vi "Arms Controller.vi"(8 "error in":errorcluster) -> ()   [LabVIEW 2017]
doc: "This VI executes continuously carrying out the current operation and responding to updates or new operations. It will often contain the timing or control code that is difficult to place directly in TeleOp. This VI generally opens all sensors and motors and isolates the rest of the robot code from knowing how the operations are carried out."
uses:
  <vilib>/Rock Robotics/WPI/Framework/Completion Status.ctl
  Arms Setpoints.ctl
  Arms Operations.ctl
  <vilib>/Rock Robotics/SystemInterfaces/DIO/FPGA_DIOPWMChannel.ctl
  <vilib>/Rock Robotics/WPI/SafetyOutput/WPI_SafetyOutputConfigMenu.ctl
  <vilib>/Rock Robotics/SystemInterfaces/DIO/FPGA_DIOChannel.ctl
  <vilib>/Rock Robotics/WPI/MotorControl/WPI_MotorControlOpen VictorSP.vi
  <vilib>/Rock Robotics/WPI/Switch/WPI_SwitchOpenLimit.vi
  <vilib>/Rock Robotics/Network Tables/NT Write Boolean.vi
panel:
  in  "Interactive Values":T1
  out "Current\nCmd":string
  in  "Buttons":cluster{"Execute Cmd":bool, "Abort Cmd":bool}
  out "Command Timing":cluster{"Start Time (ms)":u32, "Iterations":i32}
  out "Status":T3
  # "Tip: It may be helpful to observe inputs and sensor values.\nYou may also want to display tuning or debugging controls."
  # "Interactive Command: You may fill in the settings for a command\nand schedule it with the Execute button. You can observe and abort\nany command while fine tuning the code for the controller."
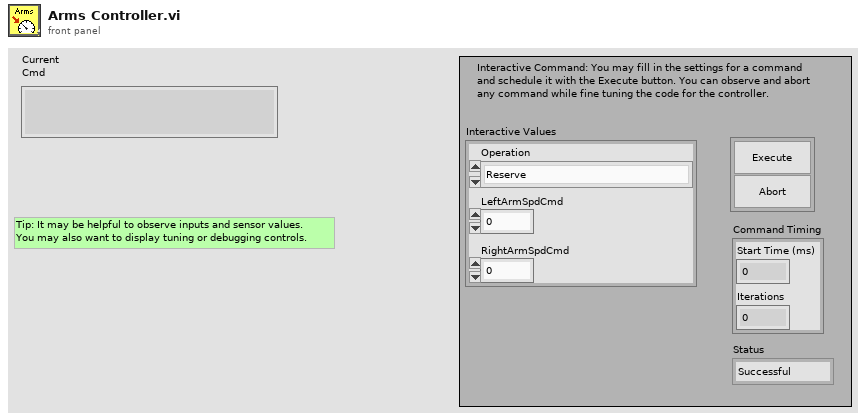
[diagram p1: front panel]
types:
  T1 = typedef "Arms Setpoints.ctl" = cluster{"Operation":T2, "LeftArmSpdCmd":dbl, "RightArmSpdCmd":dbl}
  T2 = typedef "Arms Operations.ctl" = enum16{"Reserve", "Read Current", "Immediate"}
  T3 = typedef "Completion Status.ctl" = enum16{"Successful", "Aborted", "Incomplete"}
  T4 = typedef "FPGA_DIOChannel.ctl" = enum8{"DIO 0", "DIO 1", "DIO 2", "DIO 3", "DIO 4", "DIO 5", "DIO 6", "DIO 7", "DIO 8", "DIO 9", "DIO MXP 0", "DIO MXP 1", "DIO MXP 2", "DIO MXP 3", "DIO MXP 4", "DIO MXP 5", "DIO MXP 6", "DIO MXP 7", "DIO MXP 8", "DIO MXP 9", "DIO MXP 10", "DIO MXP 11", "DIO MXP 12", "DIO MXP 13", "DIO MXP 14", "DIO MXP 15", "SPI Port CS1", "SPI Port CS2", "SPI Port CS3", "SPI Port MISO", "SPI Port MOSI", "Invalid"}
  T5 = typedef "FPGA_DIOPWMChannel.ctl" = enum8{"PWM 0", "PWM 1", "PWM 2", "PWM 3", "PWM 4", "PWM 5", "PWM 6", "PWM 7", "PWM 8", "PWM 9", "PWM MXP 0", "PWM MXP 1", "PWM MXP 2", "PWM MXP 3", "PWM MXP 4", "PWM MXP 5", "PWM MXP 6", "PWM MXP 7", "PWM MXP 8", "PWM MXP 9", "Invalid"}
  T6 = typedef "WPI_SafetyOutputConfigMenu.ctl" = enum16{"Enable", "Disable"}
  T7 = typedef "WPI_MotorControlDeviceRef.ctl" = cluster{"DeviceStatus":errorcluster, "Type":T8, "PWM":cluster{"PWM Channel":T5, "DeadBand":T9}, "CAN":cluster{"Device Number":u8, "SetOutput VI Ref":variant, "GetOutput VI Ref":variant, "Enable VI Ref":variant, "Disable VI Ref":variant, "Data":variant}, "Invert":bool, "DIO PWM":cluster{"PWM \"Enable\" Channel":T5, "DIOChannel":T4, "PWM Rate":dbl}}
  T8 = typedef "WPI_MotorControlType.ctl" = enum16{"PWM", "CAN", "DIO PWM"}
  T9 = typedef "WPI_PWMDeadband.ctl" = cluster{"Name":string, "maxPositivePwm":i32, "minPositivePwm":i32, "centerPwm":i32, "maxNegativePwm":i32, "minNegativePwm":i32, "angularRange":u16}
  T10 = typedef "WPI_SwitchDevRef.ctl" = cluster{"DevStatus":errorcluster, "DIO Channel":T4, "CntIndex":T11, "Normally Closed":bool}
  T11 = typedef "FPGA_CounterCtrSystemIndex.ctl" = enum8{"Ctr 0", "Ctr 1", "Ctr 2", "Ctr 3", "Ctr 4", "Ctr 5", "Ctr 6", "Ctr 7", "Invalid"}
  T12 = typedef "Command Status Info.ctl" = cluster{"Name":string, "Status":T3, "notifier out":T13}
  T13 = typedef "Completion Notifier.ctl" = refnum<notifier>
  T14 = cluster{"Current Command":T1, "Command Timing":cluster{"Start Time (ms)":u32, "Iterations":i32}, "Command Arguments":cluster{"Command Info":T12, "Description":string, "Default Command":T1, "queue out":refnum<queue>, "Subsystem Name":string}}
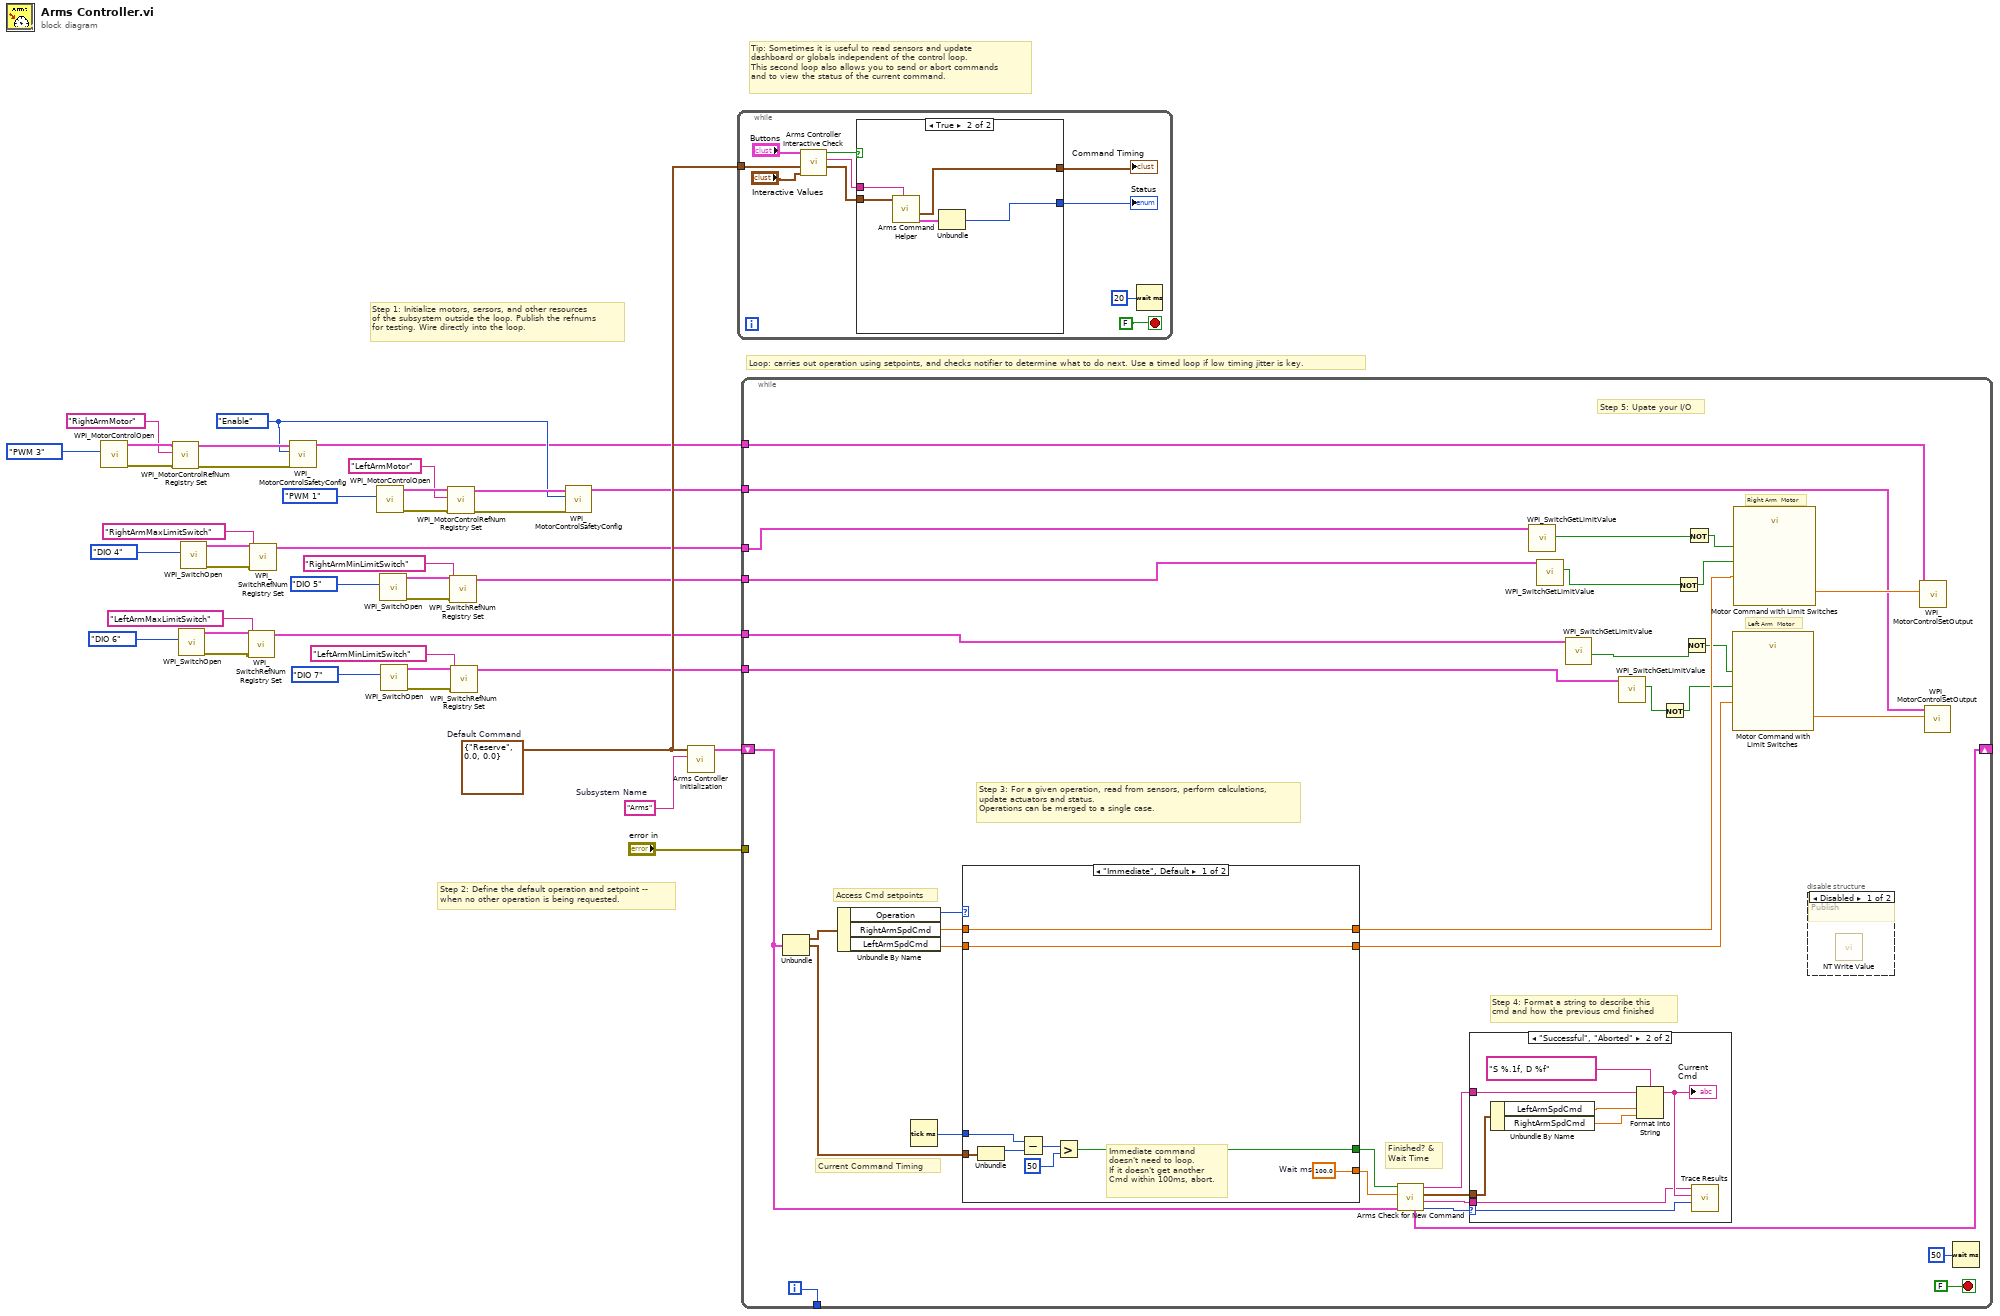
[diagram p0: block diagram]
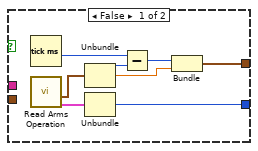
[diagram p2: hidden frame]
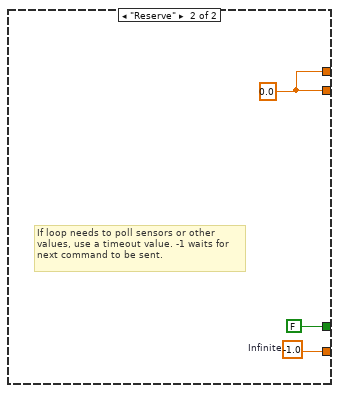
[diagram p5: hidden frame]
diagram:
  w23 = WPI_SafetyOutputConfigMenu."Enable" ("mode")
  w36 = T1 {"Operation"=enum."Reserve", "LeftArmSpdCmd"=0.0, "RightArmSpdCmd"=0.0}  # Default Command
  w37 = "Arms"  # Subsystem Name
  # "Tip: Sometimes it is useful to read sensors and update\ndashboard or globals independent of the control loop.\nThis second loop also allows you to send or abort commands\nand to view the status of the current command."
  # "Step 2: Define the default operation and setpoint --\nwhen no other operation is being requested."
  # "Step 1: Initialize motors, sersors, and other resources\nof the subsystem outside the loop. Publish the refnums\nfor testing. Wire directly into the loop."
  # "Loop: carries out operation using setpoints, and checks notifier to determine what to do next. Use a timed loop if low timing jitter is key."
  n1 = call-poly <vilib>:"WPI_MotorControlOpen.vi"("PWM Channel"=FPGA_DIOPWMChannel."PWM 3") -> ("error out"=w33:errorcluster, "MotorControlDeviceRef"=w35:T7)  [unwired: 9 in]
  n2 = call <vilib>:"WPI_MotorControlRefNum Registry Set.vi"("error in (no error)"=w33, "refnum name"="RightArmMotor", "MotorControlDevRef"=w35) -> ("error out"=w32:errorcluster, "MotorControlDevRef"=w34:T7)  [unwired: 7 in]
  n3 = call-poly <vilib>:"WPI_SwitchOpen.vi"("DIO Channel"=FPGA_DIOChannel."DIO 6") -> ("error out"=w11:errorcluster, "SwitchDevRef"=w10:T10)  [unwired: 9 in]
  n4 = call-poly <vilib>:"WPI_SwitchOpen.vi"("DIO Channel"=FPGA_DIOChannel."DIO 4") -> ("error out"=w19:errorcluster, "SwitchDevRef"=w18:T10)  [unwired: 9 in]
  n5 = call <vilib>:"WPI_SwitchRefNum Registry Set.vi"("error in (no error)"=w11, "refnum name"="LeftArmMaxLimitSwitch", "SwitchDevRef"=w10) -> ("SwitchDevRef"=w2:T10)  [unwired: 7 in, 1 out]
  n6 = call <vilib>:"WPI_SwitchRefNum Registry Set.vi"("error in (no error)"=w19, "refnum name"="RightArmMaxLimitSwitch", "SwitchDevRef"=w18) -> ("SwitchDevRef"=w3:T10)  [unwired: 7 in, 1 out]
  n7 = call <vilib>:"WPI_MotorControlSafetyConfig.vi"("error in (no error)"=w32, "mode"=w23, "MotorControlDevRef"=w34) -> ("MotorControlDevRef"=w22:T7)  [unwired: 7 in, 1 out]
  n8 = call-poly <vilib>:"WPI_MotorControlOpen.vi"("PWM Channel"=FPGA_DIOPWMChannel."PWM 1") -> ("error out"=w27:errorcluster, "MotorControlDeviceRef"=w29:T7)  [unwired: 9 in]
  n9 = call-poly <vilib>:"WPI_SwitchOpen.vi"("DIO Channel"=FPGA_DIOChannel."DIO 5") -> ("error out"=w15:errorcluster, "SwitchDevRef"=w14:T10)  [unwired: 9 in]
  n10 = call-poly <vilib>:"WPI_SwitchOpen.vi"("DIO Channel"=FPGA_DIOChannel."DIO 7") -> ("error out"=w7:errorcluster, "SwitchDevRef"=w6:T10)  [unwired: 9 in]
  n11 = call <vilib>:"WPI_MotorControlRefNum Registry Set.vi"("error in (no error)"=w27, "refnum name"="LeftArmMotor", "MotorControlDevRef"=w29) -> ("error out"=w26:errorcluster, "MotorControlDevRef"=w28:T7)  [unwired: 7 in]
  n12 = call <vilib>:"WPI_SwitchRefNum Registry Set.vi"("error in (no error)"=w15, "refnum name"="RightArmMinLimitSwitch", "SwitchDevRef"=w14) -> ("SwitchDevRef"=w4:T10)  [unwired: 7 in, 1 out]
  n13 = call <vilib>:"WPI_SwitchRefNum Registry Set.vi"("error in (no error)"=w7, "refnum name"="LeftArmMinLimitSwitch", "SwitchDevRef"=w6) -> ("SwitchDevRef"=w1:T10)  [unwired: 7 in, 1 out]
  n14 = call <vilib>:"WPI_MotorControlSafetyConfig.vi"("error in (no error)"=w26, "mode"=w23, "MotorControlDevRef"=w28) -> ("MotorControlDevRef"=w21:T7)  [unwired: 7 in, 1 out]
  n15 = call "Arms Controller Initialization.vi"("Subsystem Name"=w37, "Default Command"=w36) -> ("Current Command"=w38:T14)  [unwired: 9 in]
  n16 = while {
    tunnel: w36 -> [w46]
    stop <- FALSE stop-if-true
    n17 = call "Arms Controller Interactive Check.vi"("Interactive Command in"="Interactive Values", "Default Command"=w46, "Buttons"="Buttons") -> ("Interactive Command out"=w43:T1, "Trace String"=w44:string, "Schedule"=w45:bool)  [unwired: 6 in]
    n18 = case shown="True" w45 {
      tunnel: [w57 w62] -> w42
      tunnel: w43 -> [_ w60]
      tunnel: [w53 w58] -> w41
      tunnel: w44 -> [_ w61]
      frame False {
        n19 = Tick Count (ms)() -> (millisecond timer value=w52:u32)
        n20 = call "Read Arms Operation.vi"() -> ("Command Info"=w50:T12, "SubSystem Data"=w51:T1)  [unwired: 9 in, 1 out]
        n21 = Unbundle(w51) -> ("Operation"=w56:T2, "LeftArmSpdCmd"=w54:dbl)  [unwired: 1 out]
        n22 = Unbundle(w50) -> ("Status"=w57:T3)  [unwired: 2 out]
        n23 = Subtract(x=w52, y=w56) -> (x-y=w55:u32)
        n24 = Bundle(w55, "LeftArmSpdCmd"=w54) -> (w53:cluster{u32, "LeftArmSpdCmd":dbl})  [unwired: 1 in]
      }
      frame True {
        n25 = call "Arms Command Helper.vi"("Description"=w61, "SubSystem Data"=w60) -> ("Command Info Out"=w59:T12, "Command Timing"=w58:cluster{"Start Time (ms)":u32, "Iterations":i32})  [unwired: 7 in, 1 out]
        n26 = Unbundle(w59) -> ("Status"=w62:T3)  [unwired: 2 out]
      }
    }
    "Status" <- w42
    "Command Timing" <- w41
    n27 = Wait (ms)(milliseconds to wait=u32 20) -> ()  [unwired: 1 out]
  }
  n28 = while {
    shift-right: [w89] -> _
    shift-left: w38 -> [w82]
    tunnel: [w96] -> _
    tunnel: "error in" -> [_]
    tunnel: w22 -> [w79]
    tunnel: w21 -> [w77]
    tunnel: w4 -> [w71]
    tunnel: w3 -> [w75]
    tunnel: w2 -> [w74]
    tunnel: w1 -> [w73]
    i -> [w96]
    stop <- FALSE stop-if-true
    # "Left Arm  Motor"
    # "Right Arm  Motor"
    # "Step 5: Upate your I/O"
    # "Step 4: Format a string to describe this\ncmd and how the previous cmd finished"
    # "Current Command Timing"
    # "Access Cmd setpoints"
    # "Finished? &\nWait Time"
    # "Step 3: For a given operation, read from sensors, perform calculations,\nupdate actuators and status.\nOperations can be merged to a single case."
    n29 = Unbundle(w82) -> ("Current Command"=w95:T1, "Command Timing"=w91:cluster{"Start Time (ms)":u32, "Iterations":i32})  [unwired: 1 out]
    n30 = Unbundle By Name(w95) -> ("Operation"=w94:T2, "RightArmSpdCmd"=w93:dbl, "LeftArmSpdCmd"=w90:dbl)
    n31 = Tick Count (ms)() -> (millisecond timer value=w92:u32)
    n32 = case shown="\"Immediate\", Default" w94 {
      tunnel: [w114 w117] -> w87
      tunnel: [w108 FALSE ("ignore previous (F)")] -> w88
      tunnel: w91 -> [w110 _]
      tunnel: w93 -> [w107 _]
      tunnel: w92 -> [w109 _]
      tunnel: w90 -> [w106 _]
      tunnel: [w107 w115] -> w81
      tunnel: [w106 w115] -> w76
      frame "Immediate", Default {
        w114 = 100.0  # Wait ms
        # "Immediate command\ndoesn't need to loop.\nIf it doesn't get another\nCmd within 100ms, abort."
        n33 = Unbundle(w110) -> ("Start Time (ms)"=w113:u32)  [unwired: 1 out]
        n34 = Subtract(x=w109, y=w113) -> (x-y=w112:u32)
        n35 = Greater?(x=w112, y=u8 50 ("Left Motor")) -> (0:w108:bool)
      }
      frame "Reserve" {
        w115 = 0.0 ("RightArmSpdCmd")
        w117 = -1.0  # Infinite
        # "If loop needs to poll sensors or other\nvalues, use a timeout value. -1 waits for\nnext command to be sent."
      }
    }
    n36 = call "Arms Check for New Command.vi"("Current Command"=w82, "Wait time (ms)"=w87, "Finished?"=w88) -> ("Completion"=w83:T3, "Subsystem Name"=w84:string, "Current Command"=w85:T1, "Initial Trace String"=w86:string, "NextCommand"=w89:T14)  [unwired: 4 in]
    n37 = case shown="\"Successful\", \"Aborted\"" w83 {
      selector: w83 -> [_ w105]
      tunnel: w86 -> [_ w101]
      tunnel: w85 -> [_ w102]
      tunnel: w84 -> [_ w98]
      frame "Incomplete", Default {
        # "Continuing current command"
      }
      frame "Successful", "Aborted" {
        # "Report and setup for next command"
        n38 = Unbundle By Name(w102) -> ("LeftArmSpdCmd"=w104:dbl, "RightArmSpdCmd"=w99:dbl)
        n39 = Format Into String(format string="S %.1f, D %f", initial string=w101, w104, w99) -> (resulting string=w100:string)  [unwired: 1 in, 1 out]
        "Current\nCmd" <- w100
        n40 = call <vilib>:"Trace Results.vi"("Status of previous command"=w105, "Description"=w100, "Subsystem"=w98) -> ()  [unwired: 9 in]
      }
    }
    n41 = call <vilib>:"WPI_SwitchGetLimitValue.vi"("SwitchDevRef"=w75) -> ("Switch Pressed"=w64:bool)  [unwired: 8 in, 2 out]
    n42 = call <vilib>:"WPI_SwitchGetLimitValue.vi"("SwitchDevRef"=w71) -> ("Switch Pressed"=w66:bool)  [unwired: 8 in, 2 out]
    n43 = call <vilib>:"WPI_SwitchGetLimitValue.vi"("SwitchDevRef"=w74) -> ("Switch Pressed"=w68:bool)  [unwired: 8 in, 2 out]
    n44 = call <vilib>:"WPI_SwitchGetLimitValue.vi"("SwitchDevRef"=w73) -> ("Switch Pressed"=w70:bool)  [unwired: 8 in, 2 out]
    n45 = Not(x=w70) -> (.not. x?=w69:bool)
    n46 = Not(x=w66) -> (.not. x?=w65:bool)
    n47 = Not(x=w68) -> (.not. x?=w67:bool)
    n48 = Not(x=w64) -> (.not. x?=w63:bool)
    n49 = call "Motor Command with Limit Switches.vi"("LowLimitSwitch"=w69, "MotorCommandIn"=w76, "HighLimitSwitch"=w67) -> (0:w78:dbl)
    n50 = call "Motor Command with Limit Switches.vi"("LowLimitSwitch"=w65, "MotorCommandIn"=w81, "HighLimitSwitch"=w63) -> (0:w80:dbl)
    n51 = disable-structure shown="Disabled" {
      frame Disabled {
        # "Publish"
        n52 = call-poly <vilib>:"NT Write Value.vi"() -> ()  [unwired: 11 in, 1 out]
      }
      frame Enabled {
      }
    }
    n53 = call <vilib>:"WPI_MotorControlSetOutput.vi"("Output"=w80, "MotorControlDevRef"=w79) -> ()  [unwired: 7 in, 3 out]
    n54 = call <vilib>:"WPI_MotorControlSetOutput.vi"("Output"=w78, "MotorControlDevRef"=w77) -> ()  [unwired: 7 in, 3 out]
    n55 = Wait (ms)(milliseconds to wait=u32 50) -> ()  [unwired: 1 out]
  }
